vi "GT_BufIO.vi"(7 "Crd":i16, 8 "Typle":u16(ring) items=["MC_ENABLE"=10, "MC_CLEAR"=11, "MC_GPO"=12], 9 "doValue":u16, 10 "doMask":u16, 11 "rtn_In":cluster{"rtn":i16, "Func":string}) -> (1 "fifo":i16, 2 "Crd":i16, 3 "rtn_Out":cluster{"rtn":i16, "Func":string})   [LabVIEW 2014]
uses:
  VC6/gts.dll
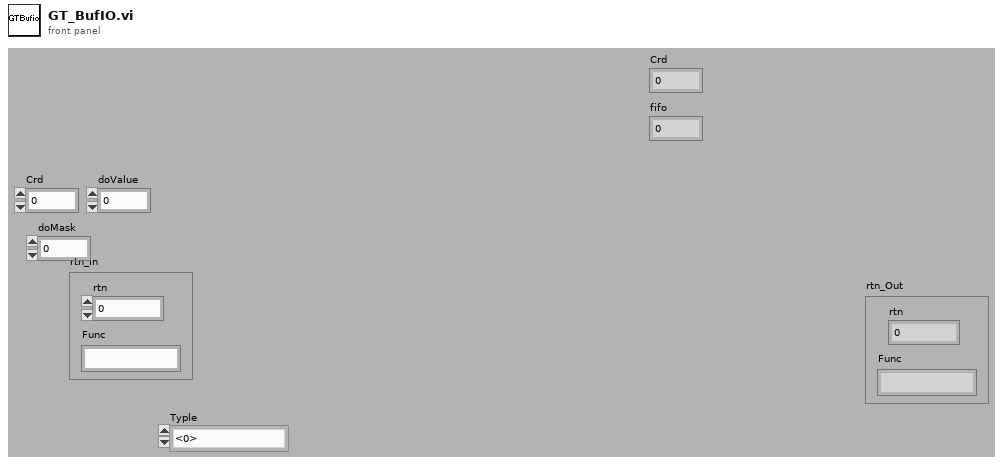
[diagram p1: front panel]
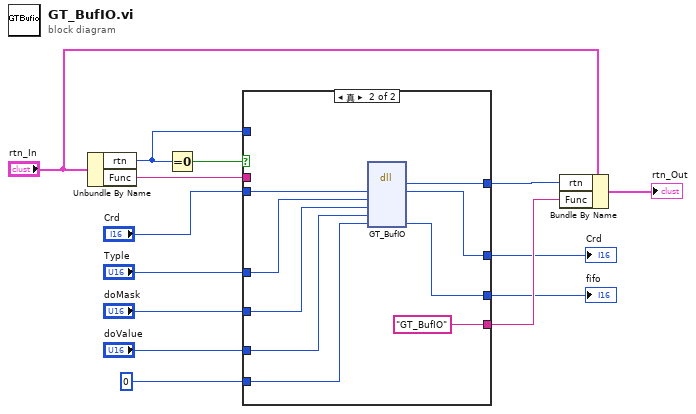
[diagram p0: block diagram]
diagram:
  n1 = Unbundle By Name("rtn_In") -> ("rtn"=w4:i16, "Func"=w3:string)
  n2 = Equal To 0?(x=w4) -> (x = 0?=w14:bool)
  n3 = case shown="真" w14 {
    tunnel: "Crd" -> [w16 w27]
    tunnel: "Typle" -> [_ w26]
    tunnel: "doMask" -> [_ w25]
    tunnel: "doValue" -> [_ w24]
    tunnel: i16 0 ("fifo") -> [w15 w23]
    tunnel: [w18 w22] -> w7
    tunnel: [w17 "GT_BufIO"] -> w5
    tunnel: w4 -> [w18 _]
    tunnel: w3 -> [w17 _]
    tunnel: [w16 w20] -> w2
    tunnel: [w15 w19] -> w1
    frame False {
    }
    frame True {
      n4 = dll-call lib="PTH2Fabs DNewGTS AC-800LWin7版源程序-20170926gts85VC6gts.dll" fn="GT_BufIO"("Crd"=w27, "doType"=w26, "doMask"=w25, "doValue"=w24, "fifo"=w23) -> ("rtn"=w22:i16, "Crd"=w20:i16, "fifo"=w19:i16)  [unwired: 6 in, 2 out]
    }
  }
  "Crd" <- w2
  "fifo" <- w1
  n5 = Bundle By Name(cluster="rtn_In", "rtn"=w7, "Func"=w5) -> (→"rtn_Out":cluster{"rtn":i16, "Func":string})
